vi "uTTA_CheckForErrors.vi"(8 "error in":errorcluster, 11 "Received":string) -> (0 "error out":errorcluster)   [LabVIEW 2021]
uses:
  <vilib>/Utility/error.llb/DialogType.ctl
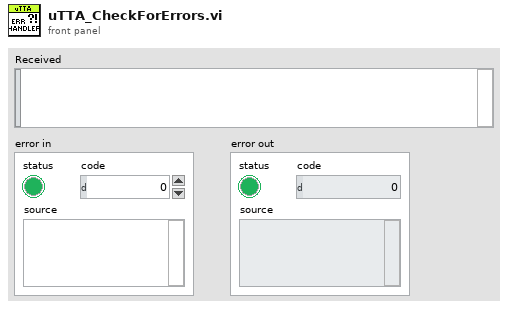
[diagram p1: front panel]
types:
  T1 = typedef "DialogType.ctl" = u16
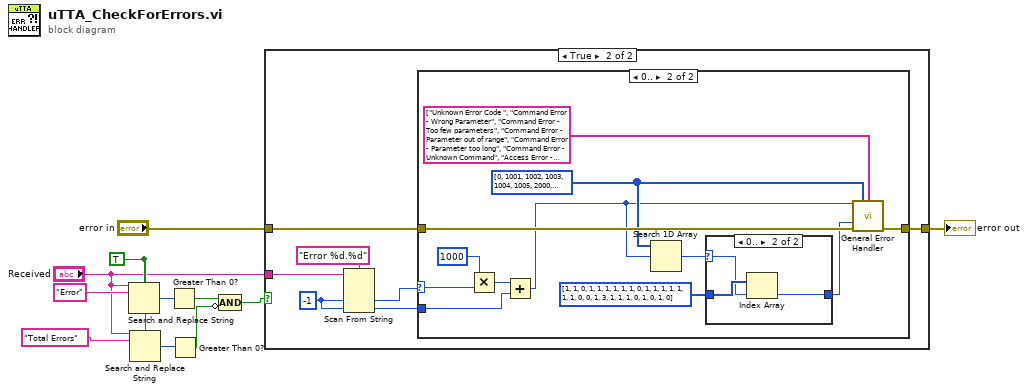
[diagram p0: block diagram]
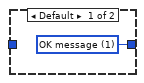
[diagram p4: hidden frame]
diagram:
  w8 = TRUE ("ignore case? (F)")
  n1 = Search and Replace String(case sensitive?=w8, input string="Received", search string="Error" ("format string")) -> (number of replacements=w4:i32)  [unwired: 5 in, 3 out]
  n2 = Search and Replace String(case sensitive?=w8, input string="Received", search string="Total Errors" ("format string")) -> (number of replacements=w5:i32)  [unwired: 5 in, 3 out]
  n3 = Greater Than 0?(x=w4) -> (x > 0?=w3:bool)
  n4 = Greater Than 0?(x=w5) -> (x > 0?=w2:bool)
  n5 = Compound Arithmetic op=AND(w3, invert w2) -> (w1:bool)
  n6 = case shown="True" w1 {
    tunnel: [w12 w19] -> w11
    tunnel: "error in" -> [w12 w18]
    tunnel: "Received" -> [_ w13]
    frame False {
    }
    frame True {
      w16 = -1 ("default value 1")
      n7 = Scan From String(format string="Error %d.%d", input string=w13, default 1=w16, default 2=w16) -> (output 1=w15:i32, output 2=w14:i32)  [unwired: 2 in, 3 out]
      n8 = case shown="0.." w15 {
        selector: w15 -> [_ w30]
        tunnel: w18 -> [w20 w28]
        tunnel: [w20 w26] -> w19
        tunnel: w14 -> [_ w32]
        frame Default {
        }
        frame 0.. {
          w22 = T1[] [1, 1, 0, 1, 1, 1, 1, 1, 1, 0, 1, 1, 1, 1, 1, 1, 1, 0, 0, 1, 3, 1, 1, 1, 0, 1, 0, 1, 0] items=["no dialog", "OK message", "continue or stop message", "OK message + warnings", "continue/stop + warnings"] ("Type of Dialog")
          w25 = i32[] [0, 1001, 1002, 1003, 1004, 1005, 2000, 2098, 2099, 3001, 3002, 3003, 3004, 3005, 3006, 4172, 4195, 4217, 4220, 4228, 4229, 4234, 4235, 4236, 4239, 4244, 4247, 4251, 4254] ("Error Codes")
          n9 = Multiply(x=1000, y=w30) -> (x*y=w29:i32)
          n10 = Add(x=w29, y=w32) -> (x+y=w24:i32)
          n11 = Search 1D Array(1D array=w25, element=w24) -> (index of element=w23:i32)  [unwired: 1 in]
          n12 = case shown="0.." w23 {
            selector: w23 -> [_ w35]
            tunnel: w22 -> [_ w36]
            tunnel: [w33 w34] -> w21
            frame Default {
              w33 = T1 1 items=["no dialog", "OK message", "continue or stop message", "OK message + warnings", "continue/stop + warnings"] ("type of dialog")
            }
            frame 0.. {
              n13 = Index Array(array=w36, index=w35) -> (element=w34:T1)
            }
          }
          n14 = call <vilib>:"General Error Handler.vi"("[error code] (0)"=w24, "[user-defined codes]"=w25, "[user-defined descriptions]"=string[] ["Unknown Error Code ", "Command Error - Wrong Parameter", "Command Error - Too few parameters", "Command Error - Parameter out of range", "Command Error - Parameter too long", "Command Error - Unknown Command", "Access Error - Measurement running", "Access Error - Measurement running", "Access Error - Command not allowed in this mode", "System Error - No SD-card installed", "System Error - File exists, can't overwrite existing files", "System Error - File not found", "System Error - Gatedriver Undervoltage", "System Error - File Write Error", "System Error - ADC Buffer Overrun", "File System Error - File System Corrupted", "File System Error - No data/attr available", "File System Error - Dir is not empty", "File System Error - File name too long", "File System Error - No space left on device", "File System Error - File too large", "File System Error - Invalid parameter", "File System Error - Entry is a dir", "File System Error - Entry is not a dir", "File System Error - Entry already exists", "File System Error - No more memory available", "File System Error - Bad file number", "File System Error - Error during device operation", "File System Error - No directory entry"] ("Error Messages"), "type of dialog (OK msg:1)"=w21, "error in (no error)"=w28) -> ("error out"=w26:errorcluster)  [unwired: 6 in, 4 out]
        }
      }
    }
  }
  "error out" <- w11
